vi "Simple UDP - Receiver Test.vi"() -> (2 "Test Passed?":bool)   [LabVIEW 2015]
doc: "The UDP protocol differs from TCP in that there is no error-checking with the packets of information that are sent, and thus no guarantee whatsoever that an intended recipient will actually receive a given piece of data.\n\nUDP does offer the ability to \"broadcast\" data across a network--simply specify an IP Address of all ones (255.255.255.255) to attempt to broadcast information network-wide. Keep in mind that routers and other network hardware will generally refuse to forward the broadcast beyond certain points, so the extent of the broadcast will in practice be limited."
panel:
  out "Iteration Count":dbl
  out "Waveform Chart":dbl(graph)
  in  "Stop":bool
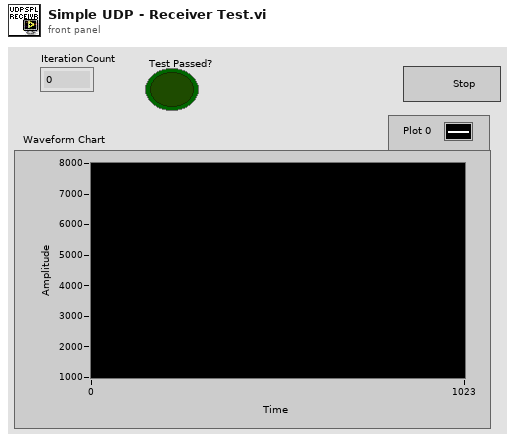
[diagram p1: front panel]
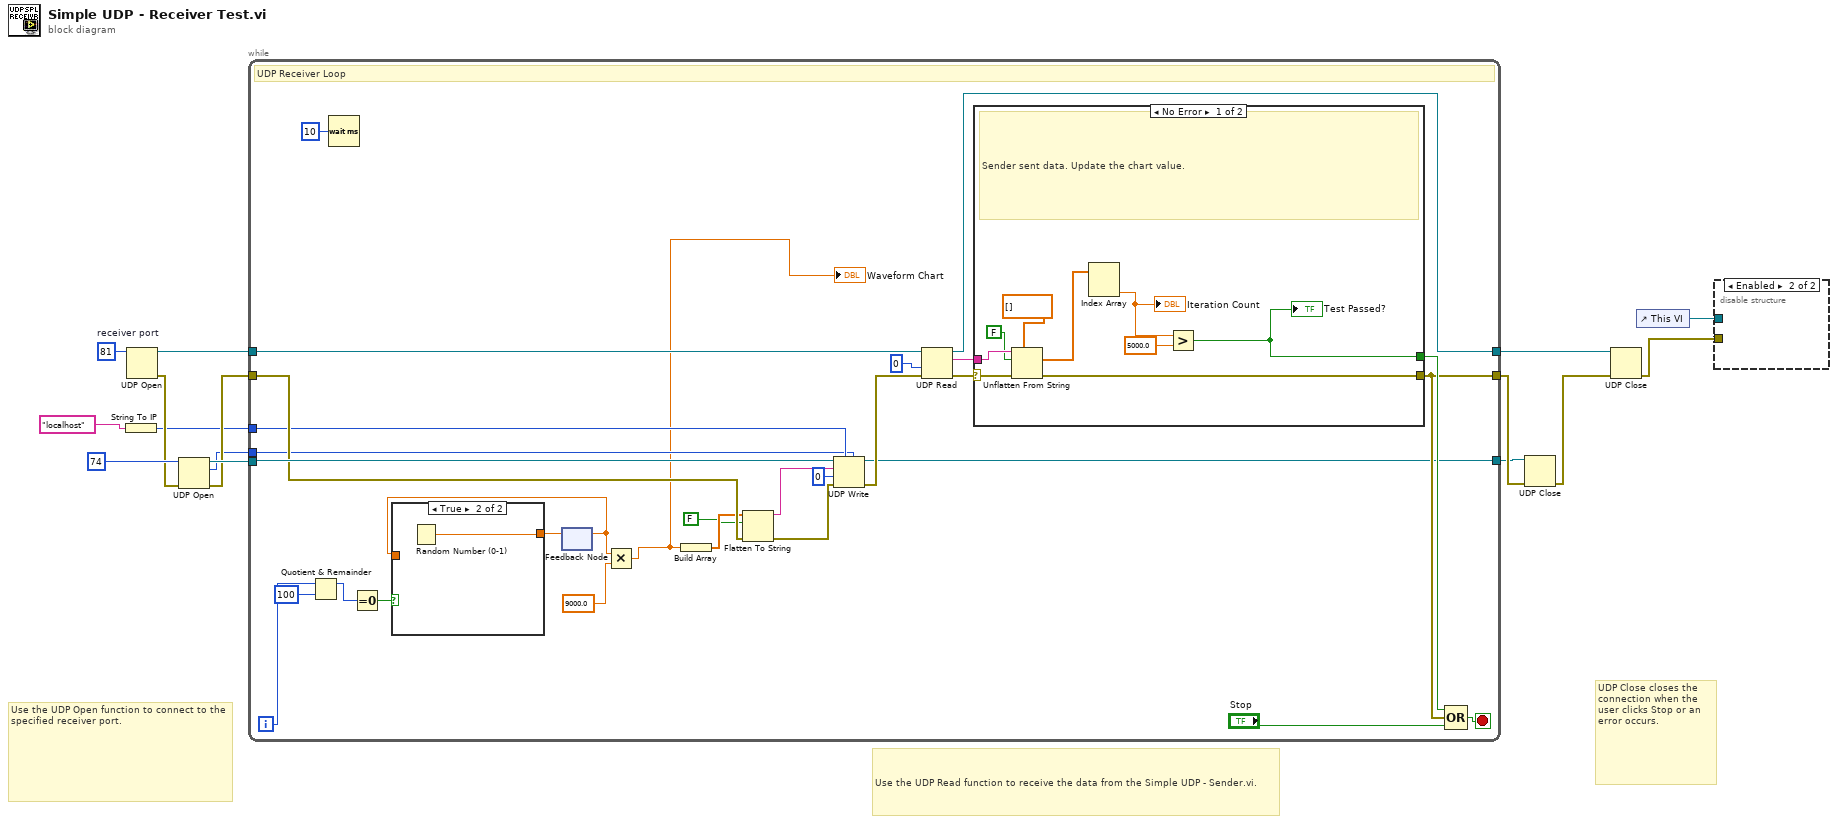
[diagram p0: block diagram]
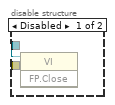
[diagram p2: hidden frame]
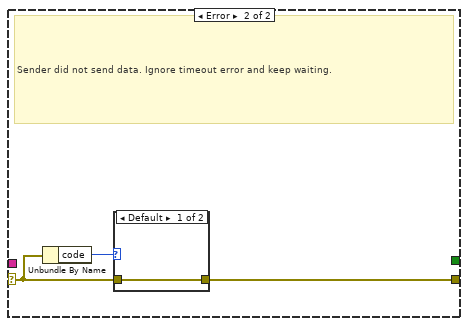
[diagram p4: hidden frame]
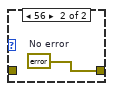
[diagram p5: hidden frame]
diagram:
  w13 = u16 81  # receiver port
  # "UDP Close closes the connection when the user clicks Stop or an error occurs."
  # "Use the UDP Open function to connect to the specified receiver port."
  # "Use the UDP Read function to receive the data from the Simple UDP - Sender.vi."
  n1 = String To IP(1:"localhost") -> (0:w2:u32)
  n2 = UDP Open(11:w13) -> (port=w14:refnum<k16>, 0:w8:errorcluster)  [unwired: 4 in, 1 out]
  n3 = UDP Open(8:w8, 11:u16 74 ("port")) -> (port=w9:refnum<k16>, 0:w7:errorcluster, 2:w1:u16)  [unwired: 3 in]
  n4 = while {
    tunnel: w14 -> [w44]
    tunnel: [w38] -> w15
    tunnel: w7 -> [w33]
    tunnel: [w36] -> w6
    tunnel: w9 -> [w35]
    tunnel: [w31] -> w4
    tunnel: w2 -> [w30]
    tunnel: w1 -> [w27]
    i -> [w25]
    stop <- w42 stop-if-true
    # "UDP Receiver Loop"
    n5 = Quotient & Remainder(x=w25, y=100) -> (x-y*floor(x/y)=w18:i32)  [unwired: 1 out]
    n6 = Wait (ms)(milliseconds to wait=u32 10) -> ()  [unwired: 1 out]
    n7 = Equal To 0?(x=w18) -> (x = 0?=w21:bool)
    n8 = feedback #1() -> (w19:dbl)  [unwired: 1 in]
    n9 = case shown="True" w21 {
      tunnel: [w45 w46] -> w20
      tunnel: w19 -> [w45 _]
      frame False {
      }
      frame True {
        n10 = Random Number (0-1)() -> (number: 0 to 1=w46:dbl)
      }
    }
    n11 = feedback-in #1(w20) -> ()
    n12 = Multiply(x=w19, y=9000.0) -> (x*y=w16:dbl)
    "Waveform Chart" <- w16
    n13 = Build Array(w16) -> (w29:dbl[])
    n14 = Flatten To String(anything=w29, prepend array or string size? (T)=FALSE, error in (no error)=w33) -> (data string=w28:string, error out=w32:errorcluster)  [unwired: 1 in, 1 out]
    n15 = UDP Write(address=w30, port or service name=w27, connection ID=w35, data in=w28, 8:w32, 9:0 ("timeout ms (25000)")) -> (error out=w34:errorcluster, 3:w31:refnum<k16>)
    n16 = UDP Read(connection ID=w44, timeout ms (25000)=0, 8:w34) -> (data out=w40:string, error out=w39:errorcluster, 3:w38:refnum<k16>)  [unwired: 3 out]
    n17 = case shown="No Error" w39 {
      selector: w39 -> [w55 w57]
      tunnel: w40 -> [w54 _]
      tunnel: [w52 w56] -> w36
      tunnel: [w48 _] -> w37
      frame No Error {
        # "Sender sent data. Update the chart value."
        n18 = Unflatten From String(type=dbl[] [], binary string=w54, data includes array or string size? (T)=FALSE, error in (no error)=w55) -> (value=w50:dbl[], error out=w52:errorcluster)  [unwired: 1 in, 1 out]
        n19 = Index Array(array=w50) -> (element #2=w47:dbl)  [unwired: 2 in, 1 out]
        "Iteration Count" <- w47
        n20 = Greater?(x=w47, y=5000.0) -> (0:w48:bool)
        "Test Passed?" <- w48
      }
      frame Error {
        # "Sender did not send data. Ignore timeout error and keep waiting."
        n21 = Unbundle By Name(w57) -> ("code"=w58:i32)
        n22 = case shown="Default" w58 {
          tunnel: w57 -> [w59 _]
          tunnel: [w59 w60] -> w56
          frame Default {
          }
          frame 56 {
            w60 = errorcluster {"status"=FALSE, "code"=0, "source"=""}  # No error
          }
        }
      }
    }
    n23 = Compound Arithmetic op=OR(w37, w36, "Stop") -> (w42:bool)
  }
  n24 = UDP Close(connection ID=w4, 8:w6) -> (error out=w5:errorcluster)  [unwired: 1 out]
  n25 = UDP Close(connection ID=w15, 8:w5) -> (error out=w12:errorcluster)  [unwired: 1 out]
  n26 = control-ref of="This VI"() -> (w11:refnum<vi>)
  n27 = disable-structure shown="Enabled" {
    disable-tunnel: w12 -> [w62 _]
    disable-tunnel: w11 -> [w61 _]
    frame Disabled {
      n28 = invoke class="VI" method="FP.Close"(reference=w61, error in=w62) -> ()  [unwired: 1 in, 3 out]
    }
    frame Enabled {
    }
  }
